vi "Create Error Entry.vi"(8 "error in (no error)":errorcluster) -> (0 "error out":errorcluster, 2 "Description":string, 3 "Code":string)   [LabVIEW 2012, in "Data Acquisition.lvlib" / "DAQ Actor.lvclass"]
uses:
  DAQ Actor.lvclass
  <vilib>/Utility/error.llb/DialogType.ctl
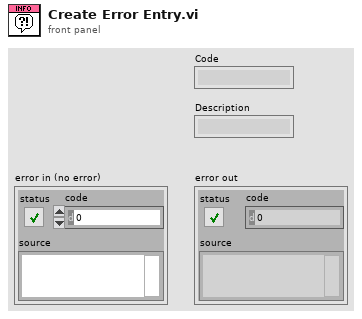
[diagram p1: front panel]
types:
  T1 = typedef "DialogType.ctl" = u16
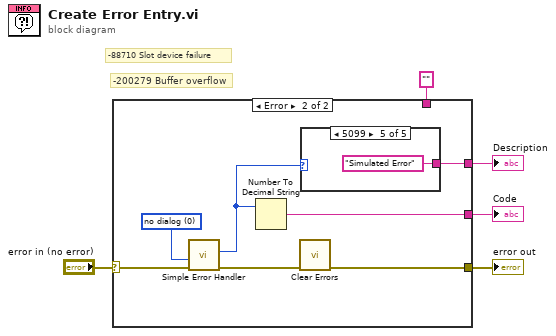
[diagram p0: block diagram]
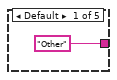
[diagram p3: hidden frame]
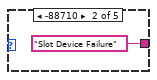
[diagram p4: hidden frame]
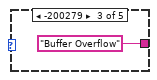
[diagram p5: hidden frame]
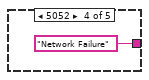
[diagram p6: hidden frame]
diagram:
  # "-88710 Slot device failure"
  # "-200279 Buffer overflow"
  n1 = case shown="Error" "error in (no error)" {
    selector: "error in (no error)" -> [w7 w10]
    tunnel: [w7 w8] -> w5
    tunnel: [w6 w13] -> w4
    tunnel: [w6 w11] -> w3
    tunnel: "" -> [w6 _]
    frame No Error {
    }
    frame Error {
      w14 = T1 0 items=["no dialog", "OK message", "continue or stop message", "OK message + warnings", "continue/stop + warnings"] ("type of dialog (OK msg:1)")
      n2 = call <vilib>:"Simple Error Handler.vi"("type of dialog (OK msg:1)"=w14, "error in (no error)"=w10) -> ("code out"=w12:i32, "error out"=w9:errorcluster)  [unwired: 3 in, 3 out]
      n3 = Number To Decimal String(number=w12) -> (decimal integer string=w11:string)  [unwired: 1 in]
      n4 = call <vilib>:"Clear Errors.vi"("error in (no error)"=w9) -> ("error out"=w8:errorcluster)  [unwired: 6 in]
      n5 = case shown="5099" w12 {
        tunnel: ["Other" "Slot Device Failure" "Buffer Overflow" "Network Failure" "Simulated Error"] -> w13
        frame Default {
        }
        frame -88710 {
        }
        frame -200279 {
        }
        frame 5052 {
        }
        frame 5099 {
        }
      }
    }
  }
  "Description" <- w4
  "error out" <- w5
  "Code" <- w3
